vi "get WFS scan derived parameters.vi"(8 "error in (no error)":errorcluster, 11 "ImagingModeSPIM in":refnum<class "ImagingModeSPIM.lvclass">) -> (0 "error out":errorcluster, 3 "ImagingModeSPIM out":refnum<class "ImagingModeSPIM.lvclass">)   [LabVIEW 2012, in "ImagingModeSPIM.lvclass"]
uses:
  ImagingModeSPIM.lvclass
  Controls/waveform_enum.ctl
  ImagingModeSPIM.lvclass/ImagingModeSPIM.ctl
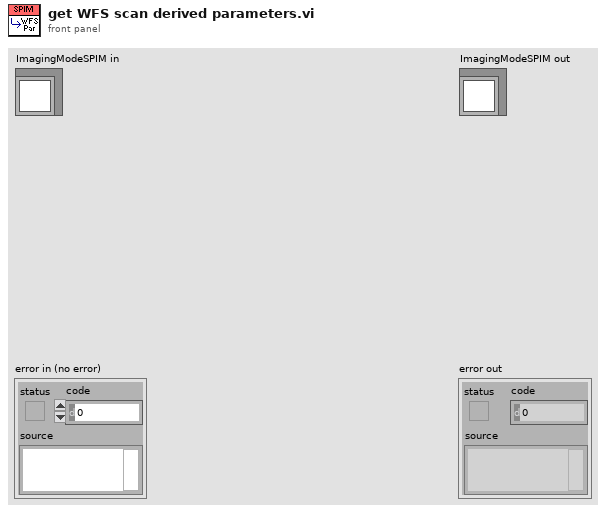
[diagram p1: front panel]
types:
  T1 = typedef "ImagingModeSPIM.lvclass/waveform_enum.ctl" = enum16{"triangular", "step", "sawtooth", "sinusodial", "skewed sawtooth"}
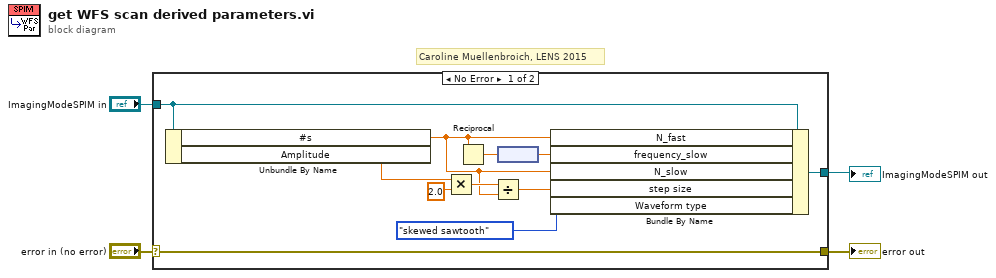
[diagram p0: block diagram]
diagram:
  # "Caroline Muellenbroich, LENS 2015"
  n1 = case shown="No Error" "error in (no error)" {
    selector: "error in (no error)" -> [w15 w17]
    tunnel: [w15 w17] -> w3
    tunnel: "ImagingModeSPIM in" -> [w14 w16]
    tunnel: [w13 w16] -> w1
    frame No Error {
      n2 = Unbundle By Name(w14) -> ("#s"=w6:dbl, "Amplitude"=w12:dbl[unit])
      n3 = Multiply(x=w12, y=2.0) -> (x*y=w11:dbl[unit])
      n4 = Reciprocal(x=w6) -> (1/x=w9:dbl)
      n5 = Divide(x=w11, y=w6) -> (x/y=w5:dbl[unit])
      n6 = node(w9) -> (w8:dbl[unit])
      n7 = Bundle By Name(cluster=w14, "N_fast"=w6, "frequency_slow"=w8, "N_slow"=w6, "step size"=w5, "Waveform type"=waveform_enum."skewed sawtooth" ("y")) -> (w13:refnum<class "ImagingModeSPIM.lvclass">)
    }
    frame Error {
    }
  }
  "error out" <- w3
  "ImagingModeSPIM out" <- w1
